vi "fftw_plan_dft_2c_1d.vi"(7 "FFTW flags":T1, 8 "error in (no error)":errorcluster, 9 "*output_data":u64, 10 "*input_data":u64, 11 "N":u32=256) -> (0 "error out":errorcluster, 1 "*output_data (copy)":u64, 2 "*input_data (copy)":u64, 3 "*plan":u64)   [LabVIEW 2020, in "FFTWDLL.lvlib"]
doc: "Plan 1D tansform from real to cplx."
uses:
  FFTWDLL.lvlib
  fftw_const_flags.ctl
  dll/libfftw3-3.dll
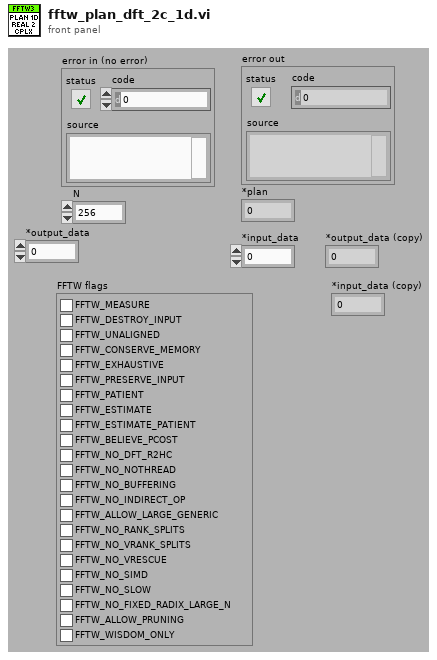
[diagram p1: front panel]
types:
  T1 = typedef "FFTWDLL.lvlib/fftw_const_flags.ctl" = cluster{"FFTW_MEASURE":bool, "FFTW_DESTROY_INPUT":bool, "FFTW_UNALIGNED":bool, "FFTW_CONSERVE_MEMORY":bool, "FFTW_EXHAUSTIVE":bool, "FFTW_PRESERVE_INPUT":bool, "FFTW_PATIENT":bool, "FFTW_ESTIMATE":bool, "FFTW_ESTIMATE_PATIENT":bool, "FFTW_BELIEVE_PCOST":bool, "FFTW_NO_DFT_R2HC":bool, "FFTW_NO_NOTHREAD":bool, "FFTW_NO_BUFFERING":bool, "FFTW_NO_INDIRECT_OP":bool, "FFTW_ALLOW_LARGE_GENERIC":bool, "FFTW_NO_RANK_SPLITS":bool, "FFTW_NO_VRANK_SPLITS":bool, "FFTW_NO_VRESCUE":bool, "FFTW_NO_SIMD":bool, "FFTW_NO_SLOW":bool, "FFTW_NO_FIXED_RADIX_LARGE_N":bool, "FFTW_ALLOW_PRUNING":bool, "FFTW_WISDOM_ONLY":bool}
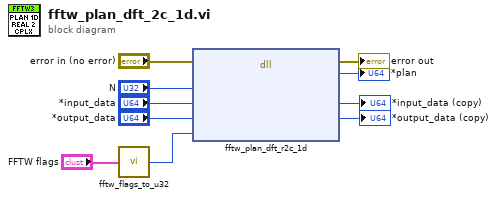
[diagram p0: block diagram]
diagram:
  n1 = call "fftw_flags_to_u32.vi"("FFTW flags"="FFTW flags") -> ("FFTW flags combined"=w4:u32)
  n2 = dll-call lib="F:/FFTWDLL/dll/libfftw3-3.dll" fn="fftw_plan_dft_r2c_1d"(error in="error in (no error)", "N"="N", "*in"="*input_data", "*out"="*output_data", "flags"=w4) -> (error out=→"error out":errorcluster, "*plan"=→"*plan":u64, "*in"=→"*input_data (copy)":u64, "*out"=→"*output_data (copy)":u64)  [unwired: 4 in, 1 out]
